vi "update.vi"(8 "error in (no error)":errorcluster, 10 "model":refnum<class "Model.lvclass">, 11 "DataStreamingState in":refnum<class "DataStreamingState.lvclass">) -> (0 "error out":errorcluster, 2 "model 2":refnum<class "Model.lvclass">, 3 "DataStreamingState out":refnum<class "DataStreamingState.lvclass">)   [LabVIEW 2013, in "DataStreamingState.lvclass"]
uses:
  DataStreamingState.lvclass
  Model/Model/Model.lvclass
  EnabledState/EnabledState.lvclass
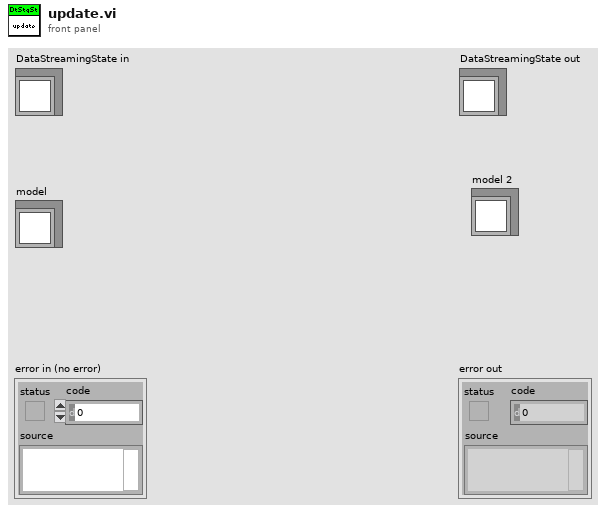
[diagram p1: front panel]
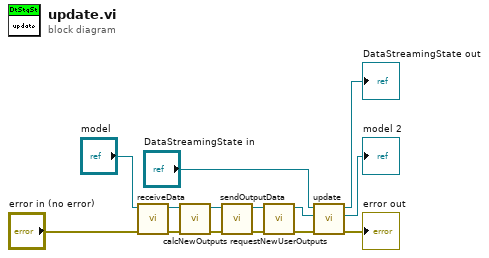
[diagram p0: block diagram]
diagram:
  n1 = call "receiveData.vi"("error in (no error)"="error in (no error)", "Model in"="model") -> ("error out"=w7:errorcluster, "Model out"=w9:refnum<class "Model.lvclass">)  [unwired: 8 in]
  n2 = call "calcNewOutputs.vi"("error in (no error)"=w7, "Model in"=w9) -> ("error out"=w6:errorcluster, "Model out"=w5:refnum<class "Model.lvclass">)  [unwired: 8 in]
  n3 = call "sendOutputData.vi"("error in (no error)"=w6, "Model in"=w5) -> ("error out"=w1:errorcluster, "Model out"=w4:refnum<class "Model.lvclass">)  [unwired: 8 in]
  n4 = call "requestNewUserOutputs.vi"("error in (no error)"=w1, "Model in"=w4) -> ("error out"=w2:errorcluster, "Model out"=w3:refnum<class "Model.lvclass">)  [unwired: 8 in]
  n5 = call-parent "update.vi"("error in (no error)"=w2, "model"=w3, "EnabledState in"="DataStreamingState in") -> ("error out"=→"error out":errorcluster, "model 2"=→"model 2":refnum<class "Model.lvclass">, "EnabledState out"=→"DataStreamingState out":refnum<class "DataStreamingState.lvclass">)  [unwired: 6 in]
